vi "Close Error Handles.vi"(8 "error in":errorcluster, 11 "Async in":refnum<class "VS Inline Async API (Express).lvclass">) -> (0 "error out":errorcluster, 3 "Async out":refnum<class "VS Inline Async API (Express).lvclass">)   [LabVIEW 2026, in "VS Inline Async API (Express).lvlib" / "VS Inline Async API (Express).lvclass"]
uses:
  VS Inline Async API (Express).lvclass
  VS Inline Async API (Express).lvclass/VS Inline Async API (Express).ctl
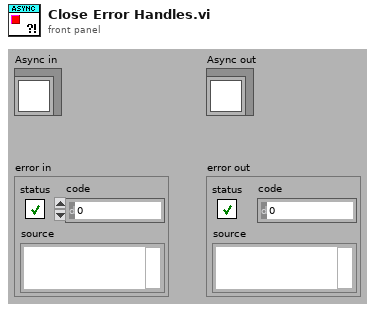
[diagram p1: front panel]
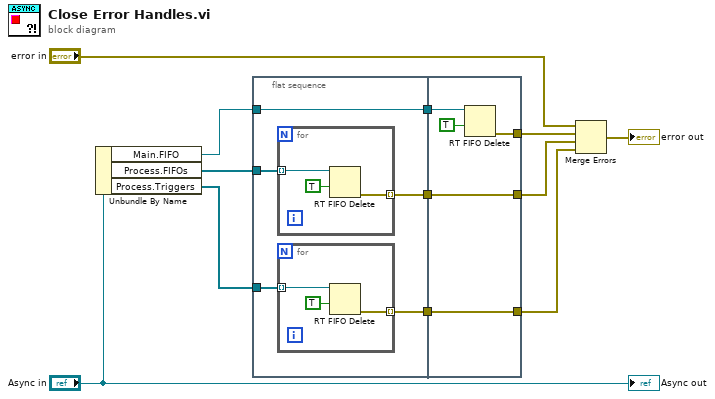
[diagram p0: block diagram]
diagram:
  n1 = Unbundle By Name("Async in") -> ("Main.FIFO"=w10:refnum<k33>, "Process.FIFOs"=w12:refnum<k33>[], "Process.Triggers"=w4:refnum<k33>[])
  n2 = flat-sequence {
    tunnel: w12 -> [w17]
    tunnel: [w16] -> w11
    tunnel: w10 -> [w16]
    tunnel: [w15] -> w7
    tunnel: w4 -> [w14]
    tunnel: [w13] -> w3
    tunnel: w11 -> [w28]
    tunnel: [w25] -> w9
    tunnel: [w27] -> w8
    tunnel: w7 -> [w27]
    tunnel: w3 -> [w24]
    tunnel: [w24] -> w2
    frame #0 {
      n3 = for {
        tunnel: w17 -> [w23] mode=indexing
        tunnel: [w21] -> w15 mode=indexing
        n4 = RT FIFO Delete(0:w23, 2:TRUE ("force destroy? (F)")) -> (11:w21:errorcluster)  [unwired: 1 in]
      }
      n5 = for {
        tunnel: w14 -> [w20] mode=indexing
        tunnel: [w18] -> w13 mode=indexing
        n6 = RT FIFO Delete(0:w20, 2:TRUE ("force destroy? (F)")) -> (11:w18:errorcluster)  [unwired: 1 in]
      }
    }
    frame #1 {
      n7 = RT FIFO Delete(0:w28, 2:TRUE ("force destroy? (F)")) -> (11:w25:errorcluster)  [unwired: 1 in]
    }
  }
  n8 = Merge Errors("error in", w9, w8, w2) -> (→"error out":errorcluster)
  "Async out" <- "Async in"
